vi "HEWH Reset Flow Meter.vi"(6 "Refnum in":T1, 7 "Use Emerson 5700":bool, 8 "error in (no error)":errorcluster, 9 "Debug":bool, 10 "Laurel Hot IP Address":string, 11 "dup VISA session in":refnum<visa-resource-name>) -> (0 "error out":errorcluster, 3 "VISA Refnum out":refnum<visa-resource-name>)   [LabVIEW 2016]
uses:
  Drivers/Laurel Meter/Type Definitions/Laurel Serial Commands.ctl
  Drivers/Emerson 5700 Transmitter/Type Definitions/Emerson 5700 Modbus Write Coils.ctl
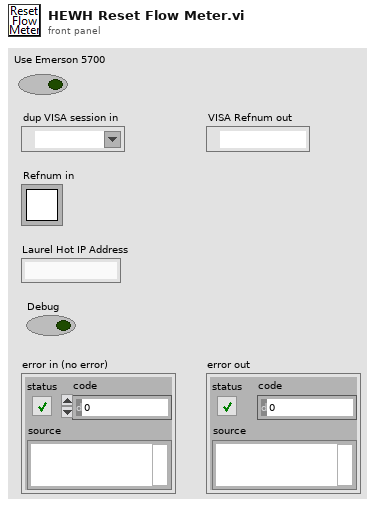
[diagram p1: front panel]
types:
  T1 = typedef "Semaphore RefNum" = refnum<k1>
  T2 = typedef "Laurel Serial Commands.ctl" = string
  T3 = enum16{"Computation Start", "Computation stop", "Reset Computation", "Clear Computation"}
  T4 = typedef "Emerson 5700 Modbus Write Coils.ctl" = u16
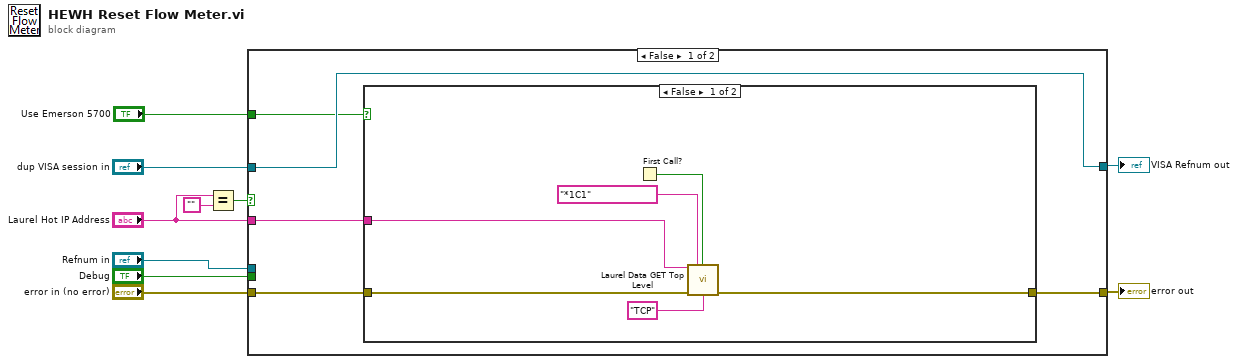
[diagram p0: block diagram]
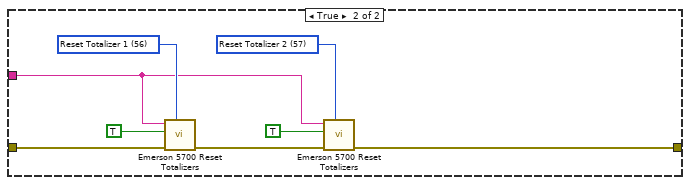
[diagram p2: hidden frame]
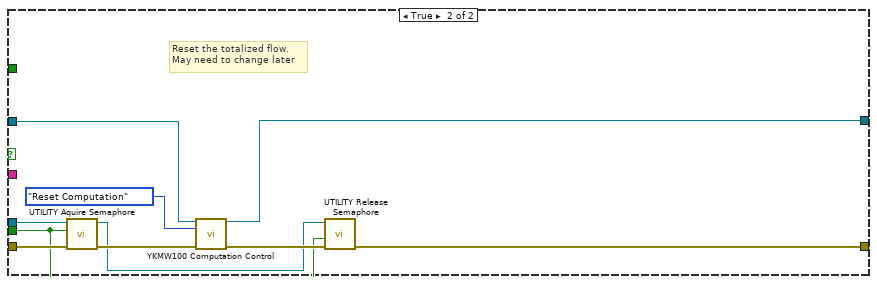
[diagram p3: hidden frame]
diagram:
  n1 = Equal?(x="Laurel Hot IP Address", y="") -> (x = y?=w3:bool)
  n2 = case shown="False" w3 {
    tunnel: "Laurel Hot IP Address" -> [w15 _]
    tunnel: "error in (no error)" -> [w14 w35]
    tunnel: [w13 w34] -> w6
    tunnel: "dup VISA session in" -> [w12 w33]
    tunnel: [w12 w32] -> w8
    tunnel: "Refnum in" -> [_ w31]
    tunnel: "Debug" -> [_ w30]
    tunnel: "Use Emerson 5700" -> [w11 _]
    frame False {
      n3 = case shown="False" w11 {
        tunnel: w15 -> [w21 w22]
        tunnel: w14 -> [w20 w29]
        tunnel: [w19 w23] -> w13
        frame False {
          n4 = First Call?() -> (First Call?: T/F=w18:bool)
          n5 = call "Laurel Data GET Top Level.vi"("Laurel IP Address"=w21, "Laurel Serial Commands"=T2 "*1C1", "First Call?"=w18, "error in (no error)"=w20, "Laurel Communication Type"="TCP") -> ("error out"=w19:errorcluster)  [unwired: 5 in, 5 out]
        }
        frame True {
          w25 = T4 57 items=["Start/Stop Inventory 1"=367, "Start/Stop Inventory 2"=368, "Start/Stop all Totalizers and Inventories"=2, "Reset all Totalizers"=3, "Reset all Inventories"=4, "Reset Totalizer 1"=56, "Reset Totalizer 2"=57] ("Reset all Totalizers. 2")
          w28 = T4 56 items=["Start/Stop Inventory 1"=367, "Start/Stop Inventory 2"=368, "Start/Stop all Totalizers and Inventories"=2, "Reset all Totalizers"=3, "Reset all Inventories"=4, "Reset Totalizer 1"=56, "Reset Totalizer 2"=57] ("Reset all Totalizers. 2")
          n6 = call "Emerson 5700 Reset Totalizers.vi"("Reset all Totalizers. 2"=w28, "Error In"=w29, "Coil"=TRUE, "address"=w22) -> ("Error Out"=w24:errorcluster)  [unwired: 7 in]
          n7 = call "Emerson 5700 Reset Totalizers.vi"("Reset all Totalizers. 2"=w25, "Error In"=w24, "Coil"=TRUE, "address"=w22) -> ("Error Out"=w23:errorcluster)  [unwired: 7 in]
        }
      }
    }
    frame True {
      # "Reset the totalized flow.\nMay need to change later"
      n8 = call "UTILITY Aquire Semaphore.vi"("error in (no error)"=w35, "Debug"=w30, "Refnum in"=w31) -> ("error out"=w38:errorcluster, "Refnum out"=w37:T1)  [unwired: 6 in, 1 out]
      n9 = call "YKMW100 Computation Control.vi"("VISA session"=w33, "Mode"=T3."Reset Computation", "error in (no error)"=w38) -> ("dup VISA session"=w32:refnum<visa-resource-name>, "error out"=w39:errorcluster)  [unwired: 11 in]
      n10 = call "UTILITY Release Semaphore.vi"("error in (no error)"=w39, "Debug"=w30, "Refnum in"=w37) -> ("error out"=w34:errorcluster)  [unwired: 8 in]
    }
  }
  "VISA Refnum out" <- w8
  "error out" <- w6
